vi "MP-Registry.vi"(6 "Action":T18 caption="Action (def: Read)", 7 "Micropulse # In":i32, 8 "error in (no error)":errorcluster, 10 "Data in":variant) -> (0 "error out":errorcluster, 2 "Micropulse Data":T2={"Instrument Type"=enum."MicroPulse 5", "Serial #"=0, "Sample Frequency"=enum."100MHz", "dt (us)"=0.0, "DOF"=enum."8-bit Mode", "Material Velocity"=1.0, "Asynch Reads"=enum."Disabled", "NUM of Tests"=0, "System Details"={"System Type"=enum."MicroPulse 5", "Serial No."=0, "Channels"={"Conv"=0, "PA"=0, "Extra"=0}, "Sample Frequency"={"Default"=0, "Actual"=0}, "Software Versions"="", "Data Output Format"={"Default"=enum."8-bit Mode", "Actual"=enum."8-bit Mode"}, "Temperatures"={"System"=0, "Processor"=0, "Slave Sys"=0, "Slave Proc"=0}, "Tx Buffer Size"=0, "System Error"="", "No. of Cards"=0, "DAC Gain"=0, "Uptimes"={"since Power"=0, "since RSTS"=0, "since SRST"=0}, "Voltages"=[], "Interface Cards"=[]}, "Gates"=[], "Encoders"=[], "CMD LUT"=variant, "Command List"=""} {"System Details"."Interface Cards"."FPGA - T" format="%.0f °C"; "System Details"."Interface Cards"."Board - T" format="%.0f °C"; "System Details"."Voltages"."Difference" format="%.2fV"; "System Details"."Voltages"."Measured" format="%.2fV"; "System Details"."Voltages"."Nominal" format="%.2fV"; "System Details"."DAC Gain" format="%.0fdB"; "System Details"."Tx Buffer Size" format="%.0fMB"; "System Details"."Temperatures"."Slave Proc" format="%.0f C"; "System Details"."Temperatures"."Slave Sys" format="%.0f C"; "System Details"."Temperatures"."Processor" format="%.0f C"; "System Details"."Temperatures"."System" format="%.0f C"; "System Details"."Sample Frequency"."Actual" format="%.0fMHz"; "System Details"."Sample Frequency"."Default" format="%.0fMHz"; "Encoders"."Encoder Filter" max=255; "Encoders"."Backlash Period (s)" min=0.0005 max=10.0 step=0.0005; "Encoders"."Multiplier" min=1 max=100000; "Encoders"."Counts/mm" min=1 max=100000; "Gates"."Insp Gates"."Max # Peaks" max=64000 step=100; "Gates"."Insp Gates"."Threshold" min=10 max=4095 step=10; "Gates"."Insp Gates"."Length (us)" min=0.0 max=96000.0 step=100.0; "Gates"."Insp Gates"."Start (us)" min=0.0 max=64000.0 step=100.0; "Gates"."Echo Gate"."Threshold" min=10 max=4095 step=10; "Gates"."Echo Gate"."Length (us)" min=0.0 max=96000.0 step=100.0; "Gates"."Echo Gate"."Start (us)" min=0.0 max=64000.0 step=100.0; "Gates"."Display Gate"."Length" min=0.0 max=64000.0 step=1000.0; "Gates"."Display Gate"."Start" min=0.0 max=64000.0 step=1000.0}, 3 "TCP config":T1={"Connection ID"=refnum, "IP address"="10.1.1.2", "host port"=1067, "OC timeout"=-1, "Read timeout"=0, "Write timeout"=0} {"Write timeout" format="%dms"; "Read timeout" format="%dms"; "OC timeout" format="%dms"}, 5 "Micropulse # Out":i32)   [LabVIEW 2026, in "MicroPulse_Driver.lvlib"]
uses:
  MicroPulse_Driver.lvlib
  MP-Registry Action-Enum.ctl
  Public/Data/Datatypes/MP-Registry Data-Cluster.ctl
  <instrlib>/MicroPulse/Public/Data/Datatypes/MP - instrument type.ctl
  Public/Data/Datatypes/MP - sample frequency.ctl
  Public/Data/Datatypes/MP - data output format.ctl
  Public/Data/Datatypes/MP - asynch read mode.ctl
  Public/Data/Datatypes/MP - general system status.ctl
  Public/Data/Datatypes/MP - interface card status.ctl
  Public/Data/Datatypes/subdatatypes/MP - Registry Gates.ctl
  Public/Data/Datatypes/MP - display gate.ctl
  Public/Data/Datatypes/MP - echo gate mode.ctl
  Public/Data/Datatypes/MP - echo gate parameters.ctl
  Public/Data/Datatypes/MP - multigate inspection gate parameters.ctl
  Public/Data/Datatypes/MP - hysteresis level.ctl
  Public/Data/Datatypes/MP - multigate mode.ctl
  Public/Data/Datatypes/MP - encoder settings.ctl
  Public/Data/Datatypes/MP - encoder type.ctl
  Public/Data/Datatypes/TCP config.ctl
panel:
  out "All Micropulse Data":T2[](array[typedef]) {"System Details"."Interface Cards"."FPGA - T" format="%.0f °C"; "System Details"."Interface Cards"."Board - T" format="%.0f °C"; "System Details"."Voltages"."Difference" format="%.2fV"; "System Details"."Voltages"."Measured" format="%.2fV"; "System Details"."Voltages"."Nominal" format="%.2fV"; "System Details"."DAC Gain" format="%.0fdB"; "System Details"."Tx Buffer Size" format="%.0fMB"; "System Details"."Temperatures"."Slave Proc" format="%.0f C"; "System Details"."Temperatures"."Slave Sys" format="%.0f C"; "System Details"."Temperatures"."Processor" format="%.0f C"; "System Details"."Temperatures"."System" format="%.0f C"; "System Details"."Sample Frequency"."Actual" format="%.0fMHz"; "System Details"."Sample Frequency"."Default" format="%.0fMHz"; "Encoders"."Encoder Filter" max=255; "Encoders"."Backlash Period (s)" min=0.0005 max=10.0 step=0.0005; "Encoders"."Multiplier" min=1 max=100000; "Encoders"."Counts/mm" min=1 max=100000; "Gates"."Insp Gates"."Max # Peaks" max=64000 step=100; "Gates"."Insp Gates"."Threshold" min=10 max=4095 step=10; "Gates"."Insp Gates"."Length (us)" min=0.0 max=96000.0 step=100.0; "Gates"."Insp Gates"."Start (us)" min=0.0 max=64000.0 step=100.0; "Gates"."Echo Gate"."Threshold" min=10 max=4095 step=10; "Gates"."Echo Gate"."Length (us)" min=0.0 max=96000.0 step=100.0; "Gates"."Echo Gate"."Start (us)" min=0.0 max=64000.0 step=100.0; "Gates"."Display Gate"."Length" min=0.0 max=64000.0 step=1000.0; "Gates"."Display Gate"."Start" min=0.0 max=64000.0 step=1000.0}
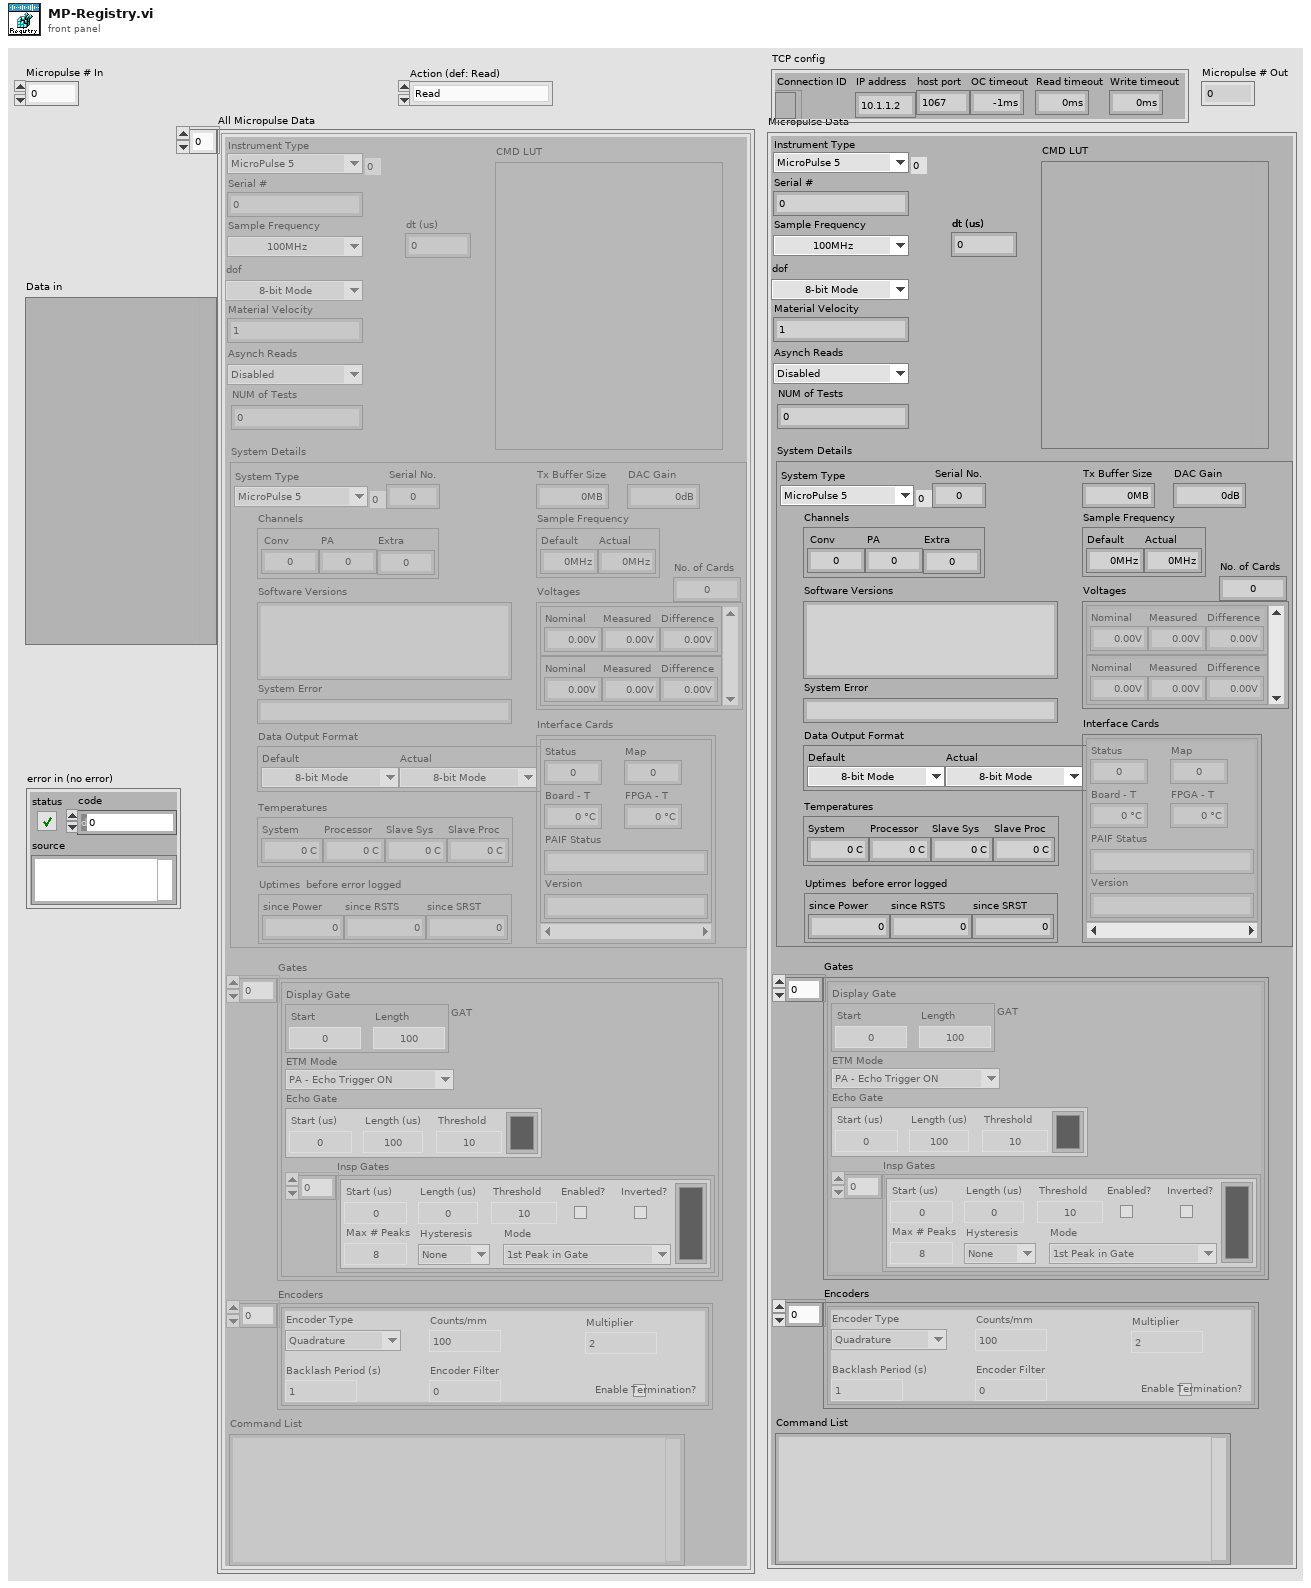
[diagram p1: front panel]
types:
  T1 = typedef "MicroPulse_Driver.lvlib/TCP config.ctl" = cluster{"Connection ID":refnum<k5>, "IP address":string, "host port":u16, "OC timeout":i32, "Read timeout":i32, "Write timeout":i32}
  T2 = typedef "MicroPulse_Driver.lvlib/MP-Registry Data-Cluster.ctl" = cluster{"Instrument Type":T3, "Serial #":u64, "Sample Frequency":T4, "dt (us)":dbl, "DOF":T5, "Material Velocity":dbl, "Asynch Reads":T6, "NUM of Tests":u32, "System Details":T7, "Gates":T9[], "Encoders":T16[], "CMD LUT":variant, "Command List":string}
  T3 = typedef "MicroPulse_Driver.lvlib/MP - instrument type.ctl" = enum16{"MicroPulse 5", "LT1", "LT2", "LTPA", "MPLT", "MicroPulse 6", "PipeScanner", "<MicroPulse>", "Micropulse 4", "Simulated Data"}
  T4 = typedef "MicroPulse_Driver.lvlib/MP - sample frequency.ctl" = enum16{"Use Default", "200MHz (LT2 only)", "100MHz", "50MHz", "25MHz", "10MHz"}
  T5 = typedef "MicroPulse_Driver.lvlib/MP - data output format.ctl" = enum16{"", "8-bit Mode", "10-bit Mode", "12-bit Mode", "16-bit Mode", "8-bit Log Mode", "12-bit Packed Mode"}
  T6 = typedef "MicroPulse_Driver.lvlib/MP - asynch read mode.ctl" = enum16{"Disabled", "Enabled"}
  T7 = typedef "MicroPulse_Driver.lvlib/MP - general system status.ctl" = cluster{"System Type":T3, "Serial No.":u64, "Channels":cluster{"Conv":u8, "PA":u16, "Extra":u32}, "Sample Frequency":cluster{"Default":u8, "Actual":u8}, "Software Versions":string, "Data Output Format":cluster{"Default":T5, "Actual":T5}, "Temperatures":cluster{"System":u8, "Processor":u8, "Slave Sys":u8, "Slave Proc":u8}, "Tx Buffer Size":u32, "System Error":string, "No. of Cards":u8, "DAC Gain":i16, "Uptimes":cluster{"since Power":u32, "since RSTS":u32, "since SRST":u32}, "Voltages":cluster{"Nominal":dbl, "Measured":dbl, "Difference":dbl}[], "Interface Cards":T8[]}
  T8 = typedef "MicroPulse_Driver.lvlib/MP - interface card status.ctl" = cluster{"Status":u8, "Map":u8, "Board - T":u8, "FPGA - T":u8, "PAIF Status":string, "Version":string}
  T9 = typedef "MicroPulse_Driver.lvlib/MP - Registry Gates.ctl" = cluster{"Display Gate":T10, "ETM Mode":T11, "Echo Gate":T12, "Insp Gates":T13[]}
  T10 = typedef "MicroPulse_Driver.lvlib/MP - display gate.ctl" = cluster{"Start":dbl, "Length":dbl}
  T11 = typedef "MicroPulse_Driver.lvlib/MP - echo gate mode.ctl" = enum16{"Echo Trigger OFF", "Echo Gate Display Mode", "Echo Trigger ON", "Multi Gate or FMC Mode", "Reserved", "PA - Echo Trigger ON"}
  T12 = typedef "MicroPulse_Driver.lvlib/MP - echo gate parameters.ctl" = cluster{"Start (us)":dbl, "Length (us)":dbl, "Threshold":u16, "Colour":u32}
  T13 = typedef "MicroPulse_Driver.lvlib/MP - multigate inspection gate parameters.ctl" = cluster{"Start (us)":dbl, "Length (us)":dbl, "Threshold":u16, "Enabled?":bool, "Max # Peaks":u16, "Hysteresis":T14, "Mode":T15, "Inverted?":bool, "Colour ":u32}
  T14 = typedef "MicroPulse_Driver.lvlib/MP - hysteresis level.ctl" = enum16{"None", "3dB", "6dB", "9dB", "12dB"}
  T15 = typedef "MicroPulse_Driver.lvlib/MP - multigate mode.ctl" = enum16{"1st Peak in Gate", "Largest Peak In Gate", "All Peaks In Gate", "1st Threshold Crossing"}
  T16 = typedef "MicroPulse_Driver.lvlib/MP - encoder settings.ctl" = cluster{"Encoder Type":T17, "Counts/mm":u32, "Enable Termination?":bool, "Multiplier":u32, "Backlash Period (s)":dbl, "Encoder Filter":u32}
  T17 = typedef "MicroPulse_Driver.lvlib/MP - encoder type.ctl" = enum16{"Quadrature", "Step/Direction"}
  T18 = typedef "MicroPulse_Driver.lvlib/MP-Registry Action-Enum.ctl" = enum16{"Read", "Add Test", "Add Command", "Add Gate Command", "Add Encoder Command", "Clear Command  List", "Set Registry", "Set System Details", "Set DOF", "Set Velocity", "Disable Asynch Reads", "Enable Asynch Reads", "Add Connection", "Disconnect", "Shutdown"}
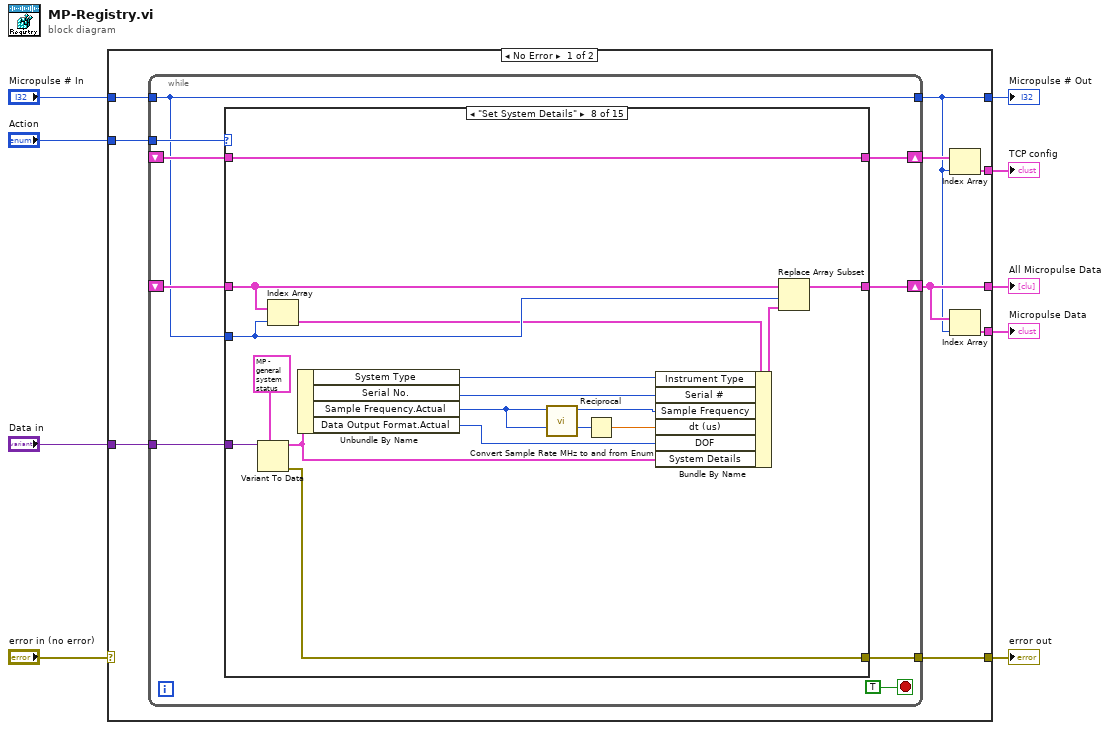
[diagram p0: block diagram]
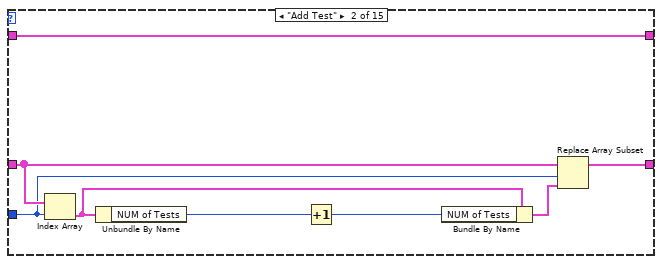
[diagram p3: hidden frame]
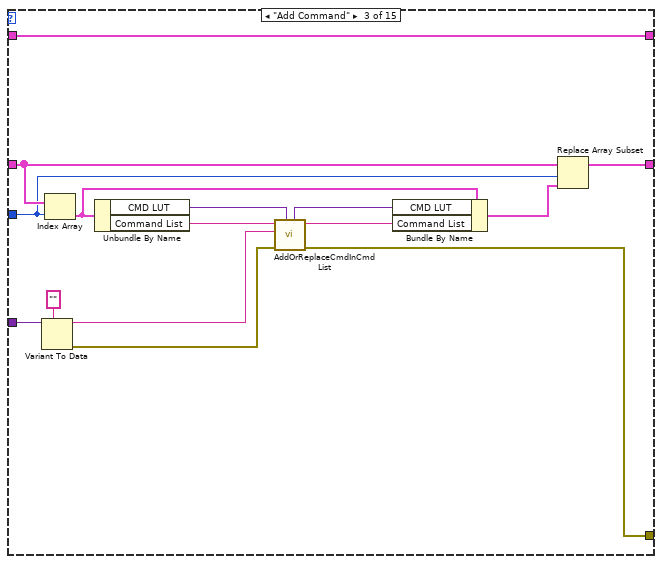
[diagram p4: hidden frame]
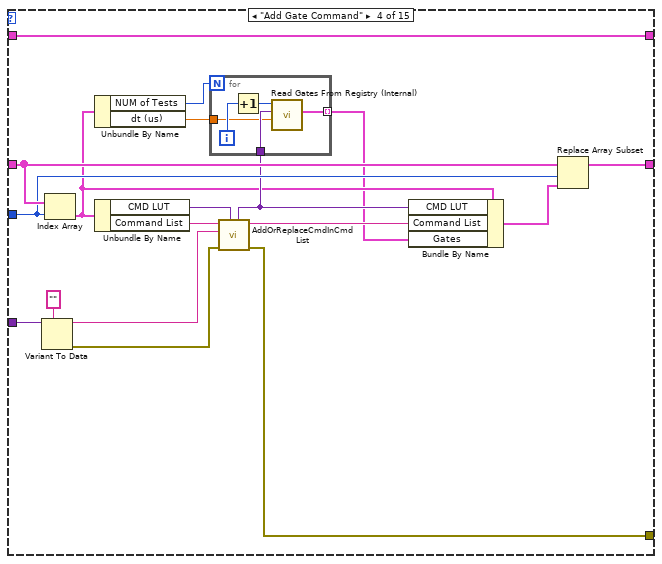
[diagram p5: hidden frame]
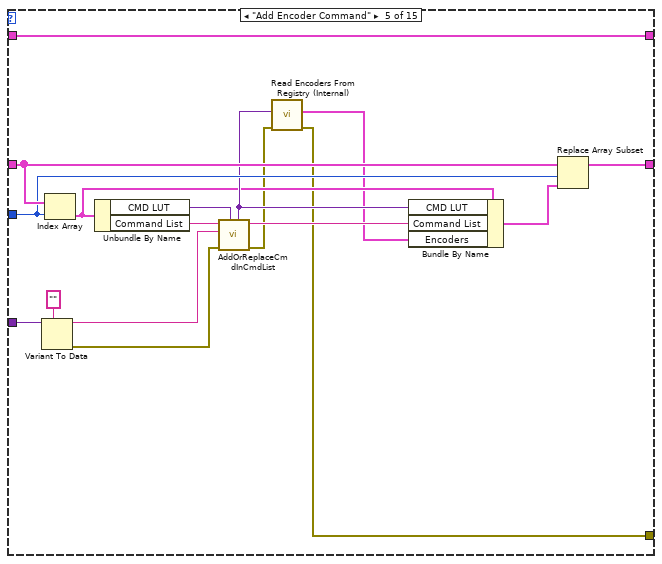
[diagram p6: hidden frame]
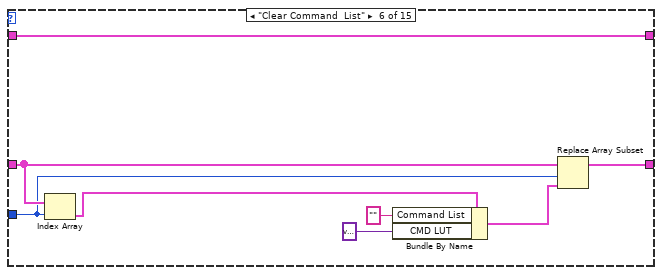
[diagram p7: hidden frame]
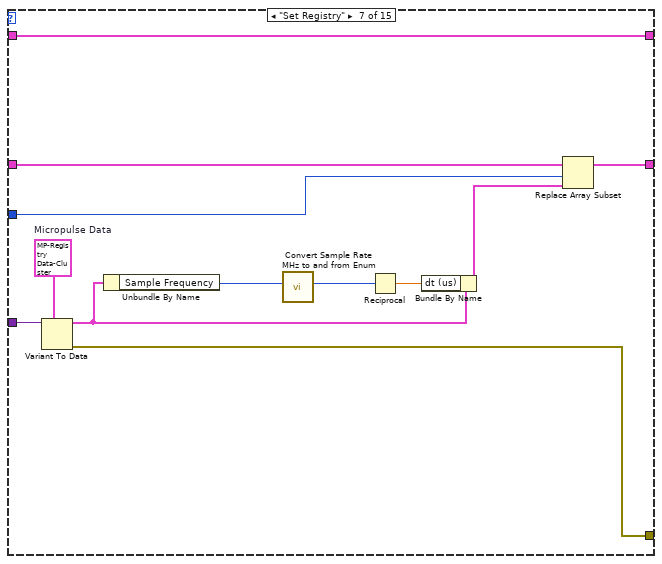
[diagram p8: hidden frame]
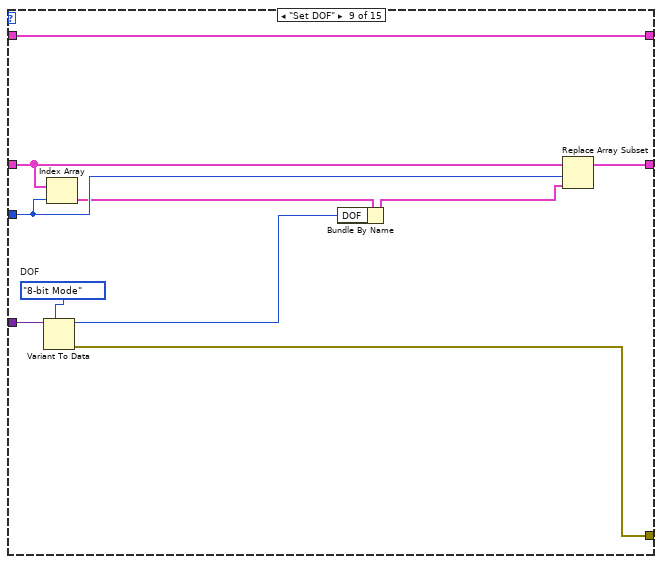
[diagram p9: hidden frame]
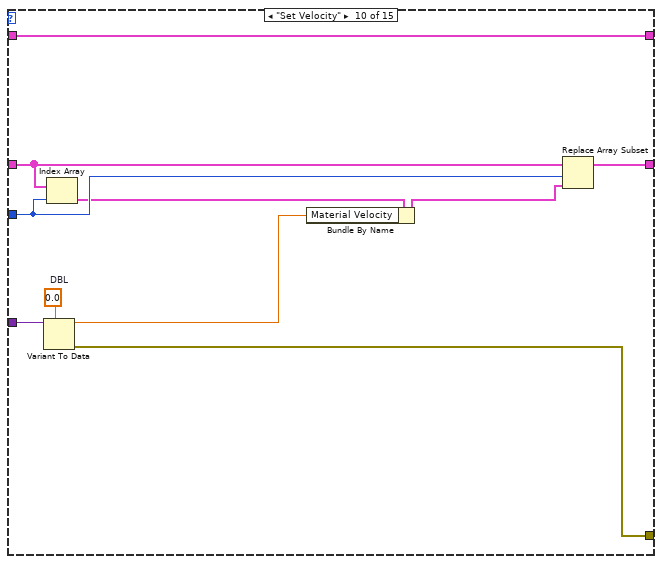
[diagram p10: hidden frame]
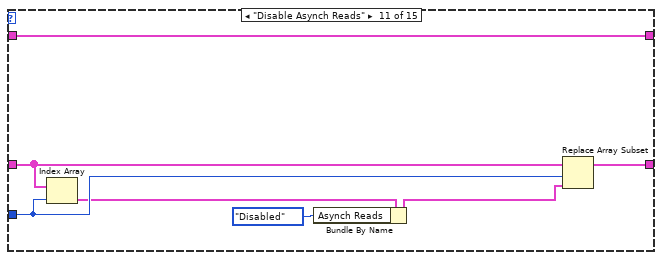
[diagram p11: hidden frame]
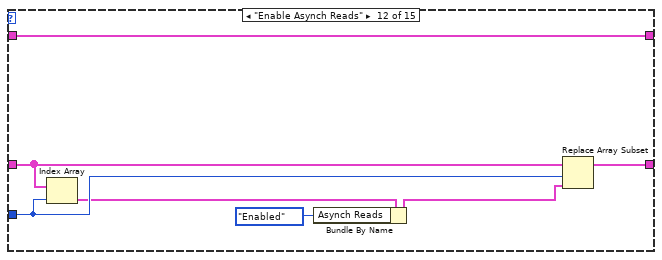
[diagram p12: hidden frame]
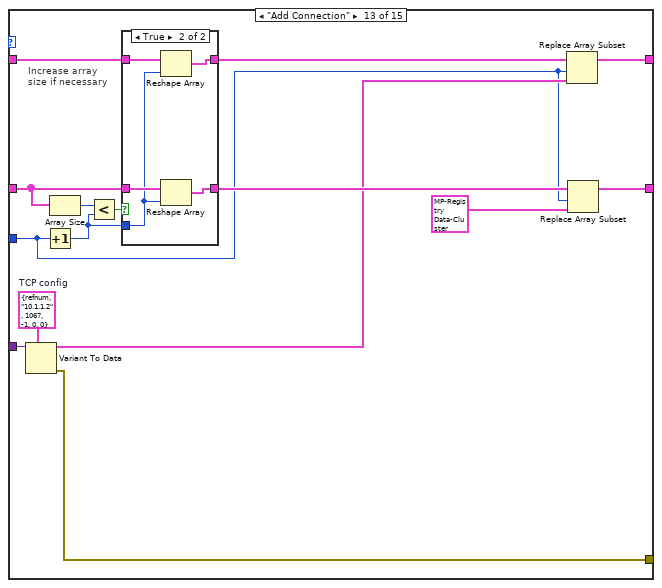
[diagram p13: hidden frame]
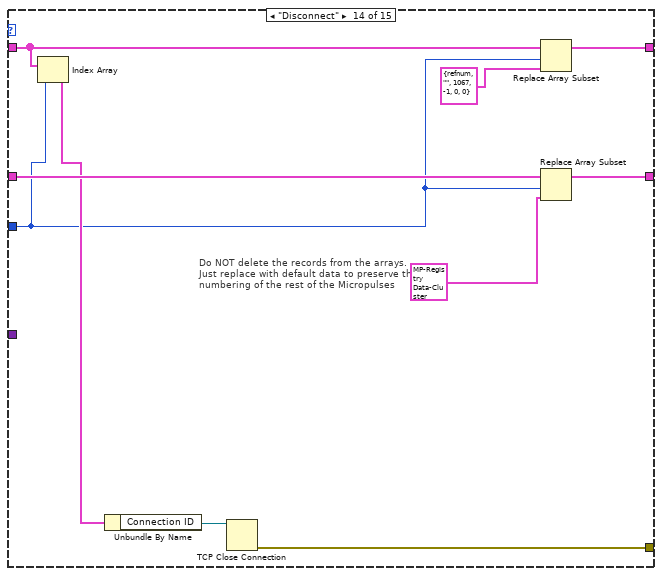
[diagram p15: hidden frame]
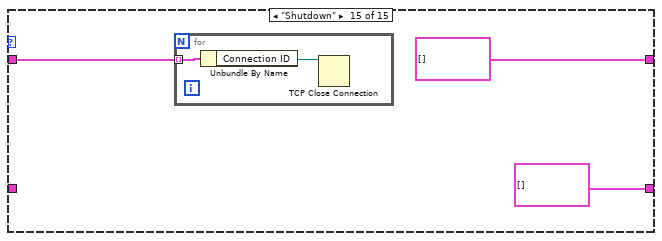
[diagram p16: hidden frame]
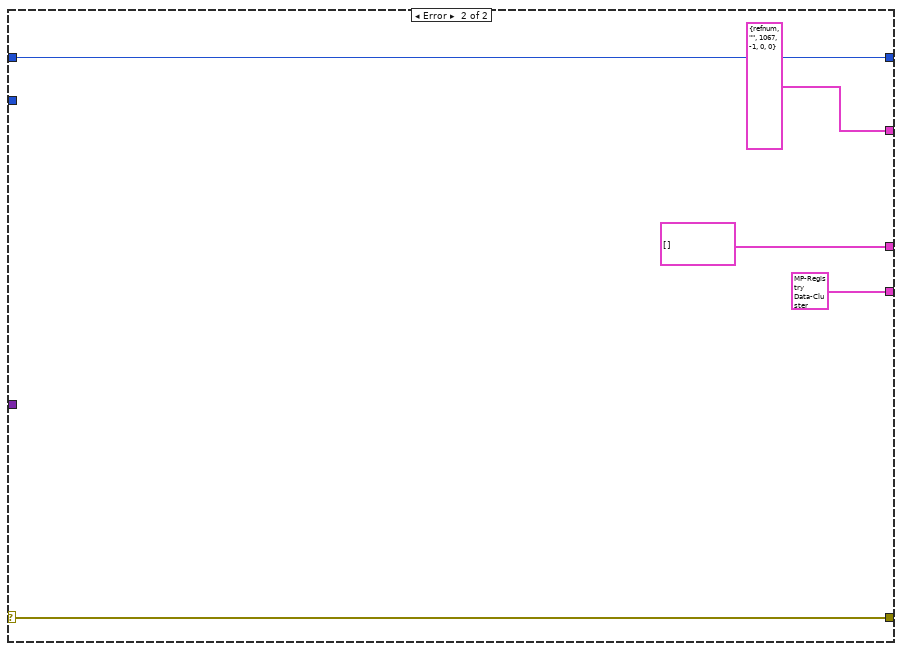
[diagram p17: hidden frame]
diagram:
  n1 = case shown="No Error" "error in (no error)" {
    selector: "error in (no error)" -> [_ w204]
    tunnel: [w12 w204] -> w8
    tunnel: "Action" -> [w18 _]
    tunnel: "Micropulse # In" -> [w16 w203]
    tunnel: [w10 w203] -> w5
    tunnel: [w15 T1 {"Connection ID"=refnum, "IP address"="", "host port"=1067, "OC timeout"=-1, "Read timeout"=0, "Write timeout"=0} ("TCP config")] -> w1
    tunnel: [w14 T2 {"Instrument Type"=enum."MicroPulse 5", "Serial #"=0, "Sample Frequency"=enum."100MHz", "dt (us)"=0.0, "DOF"=enum."8-bit Mode", "Material Velocity"=1.0, "Asynch Reads"=enum."Disabled", "NUM of Tests"=0, "System Details"={"System Type"=enum."MicroPulse 5", "Serial No."=0, "Channels"={"Conv"=0, "PA"=0, "Extra"=0}, "Sample Frequency"={"Default"=0, "Actual"=0}, "Software Versions"="", "Data Output Format"={"Default"=enum."8-bit Mode", "Actual"=enum."8-bit Mode"}, "Temperatures"={"System"=0, "Processor"=0, "Slave Sys"=0, "Slave Proc"=0}, "Tx Buffer Size"=0, "System Error"="", "No. of Cards"=0, "DAC Gain"=0, "Uptimes"={"since Power"=0, "since RSTS"=0, "since SRST"=0}, "Voltages"=[], "Interface Cards"=[]}, "Gates"=[], "Encoders"=[], "CMD LUT"=variant, "Command List"=""} ("Micropulse Data")] -> w4
    tunnel: "Data in" -> [w13 _]
    tunnel: [w11 T2[] [] ("Array")] -> w2
    frame No Error {
      n2 = while {
        shift-right: [w22] -> w11
        shift-left: _ -> [w25]
        tunnel: w18 -> [w26]
        tunnel: w16 -> [w21]
        shift-right: [w23] -> w17
        shift-left: _ -> [w24]
        tunnel: [w21] -> w10
        tunnel: w13 -> [w20]
        tunnel: [w19] -> w12
        stop <- TRUE stop-if-true
        n3 = case shown="\"Set System Details\"" w26 {
          tunnel: w21 -> [_ w34 w48 w66 w88 w97 w107 w122 w132 w143 w152 w159 w163 w185 _]
          tunnel: w25 -> [w28 w35 w50 w68 w90 w98 w111 w123 w133 w144 w153 w160 w172 w193 _]
          tunnel: w24 -> [w29 w37 w52 w70 w92 w100 w112 w128 w138 w148 w155 w162 w175 w189 w197]
          tunnel: [w29 w37 w52 w70 w92 w100 w112 w128 w138 w148 w155 w162 w168 w194 T1[] [] ("Array")] -> w23
          tunnel: [w28 w36 w51 w69 w91 w99 w110 w127 w137 w147 w154 w161 w167 w192 T2[] [] ("Array")] -> w22
          tunnel: w20 -> [_ _ w46 w64 w86 _ w109 w126 w136 w146 _ _ w170 _ _]
          tunnel: [_ _ w40 w59 w76 _ w106 w116 w134 w145 _ _ w166 w186 _] -> w19
          frame "Read", Default {
          }
          frame "Add Test" {
            n4 = Index Array(array=w35, index=w34) -> (element=w32:T2)
            n5 = Unbundle By Name(w32) -> ("NUM of Tests"=w31:u32)
            n6 = Increment(x=w31) -> (x+1=w30:u32)
            n7 = Bundle By Name(cluster=w32, "NUM of Tests"=w30) -> (w33:T2)
            n8 = Replace Array Subset(array=w35, new element=w33, index=w34) -> (w36:T2[])
          }
          frame "Add Command" {
            n9 = Variant To Data(type="", Variant=w46) -> (data=w44:string, error out=w41:errorcluster)  [unwired: 1 in]
            n10 = Index Array(array=w50, index=w48) -> (element=w42:T2)
            n11 = Unbundle By Name(w42) -> ("CMD LUT"=w39:variant, "Command List"=w49:string)
            n12 = call "AddOrReplaceCmdInCmdList.vi"("CMD LUT in"=w39, "error in (no error)"=w41, "New Command(s)"=w44, "Command List In"=w49) -> ("error out"=w40:errorcluster, "Command List Out"=w47:string, "CMD LUT out"=w38:variant)  [unwired: 5 in]
            n13 = Bundle By Name(cluster=w42, "CMD LUT"=w38, "Command List"=w47) -> (w43:T2)
            n14 = Replace Array Subset(array=w50, new element=w43, index=w48) -> (w51:T2[])
          }
          frame "Add Gate Command" {
            n15 = Variant To Data(type="", Variant=w64) -> (data=w62:string, error out=w60:errorcluster)  [unwired: 1 in]
            n16 = Index Array(array=w68, index=w66) -> (element=w56:T2)
            n17 = Unbundle By Name(w56) -> ("NUM of Tests"=w53:u32, "dt (us)"=w55:dbl)
            n18 = Unbundle By Name(w56) -> ("CMD LUT"=w58:variant, "Command List"=w67:string)
            n19 = call "AddOrReplaceCmdInCmdList.vi"("CMD LUT in"=w58, "error in (no error)"=w60, "New Command(s)"=w62, "Command List In"=w67) -> ("error out"=w59:errorcluster, "Command List Out"=w65:string, "CMD LUT out"=w57:variant)  [unwired: 5 in]
            n20 = for {
              N: w53 -> [_]
              tunnel: w57 -> [w73]
              tunnel: w55 -> [w72]
              tunnel: [w71] -> w54 mode=indexing
              i -> [w75]
              n21 = Increment(x=w75) -> (x+1=w74:i32)
              n22 = call "Read Gates From Registry (Internal).vi"("dt (us)"=w72, "CMD LUT"=w73, "Test No."=w74) -> ("Gates"=w71:T9)  [unwired: 7 in, 1 out]
            }
            n23 = Bundle By Name(cluster=w56, "CMD LUT"=w57, "Command List"=w65, "Gates"=w54) -> (w61:T2)
            n24 = Replace Array Subset(array=w68, new element=w61, index=w66) -> (w69:T2[])
          }
          frame "Add Encoder Command" {
            n25 = Variant To Data(type="", Variant=w86) -> (data=w84:string, error out=w82:errorcluster)  [unwired: 1 in]
            n26 = Index Array(array=w90, index=w88) -> (element=w79:T2)
            n27 = Unbundle By Name(w79) -> ("CMD LUT"=w81:variant, "Command List"=w89:string)
            n28 = call "AddOrReplaceCmdInCmdList.vi"("CMD LUT in"=w81, "error in (no error)"=w82, "New Command(s)"=w84, "Command List In"=w89) -> ("error out"=w77:errorcluster, "Command List Out"=w87:string, "CMD LUT out"=w80:variant)  [unwired: 5 in]
            n29 = call "Read Encoders From Registry (Internal).vi"("error in (no error)"=w77, "CMD LUT"=w80) -> ("error out"=w76:errorcluster, "Encoders"=w78:T16[])  [unwired: 8 in]
            n30 = Bundle By Name(cluster=w79, "CMD LUT"=w80, "Command List"=w87, "Encoders"=w78) -> (w83:T2)
            n31 = Replace Array Subset(array=w90, new element=w83, index=w88) -> (w91:T2[])
          }
          frame "Clear Command  List" {
            n32 = Index Array(array=w98, index=w97) -> (element=w95:T2)
            n33 = Bundle By Name(cluster=w95, "Command List"="", "CMD LUT"=variant) -> (w96:T2)
            n34 = Replace Array Subset(array=w98, new element=w96, index=w97) -> (w99:T2[])
          }
          frame "Set Registry" {
            w108 = T2 {"Instrument Type"=enum."MicroPulse 5", "Serial #"=0, "Sample Frequency"=enum."100MHz", "dt (us)"=0.0, "DOF"=enum."8-bit Mode", "Material Velocity"=1.0, "Asynch Reads"=enum."Disabled", "NUM of Tests"=0, "System Details"={"System Type"=enum."MicroPulse 5", "Serial No."=0, "Channels"={"Conv"=0, "PA"=0, "Extra"=0}, "Sample Frequency"={"Default"=0, "Actual"=0}, "Software Versions"="", "Data Output Format"={"Default"=enum."8-bit Mode", "Actual"=enum."8-bit Mode"}, "Temperatures"={"System"=0, "Processor"=0, "Slave Sys"=0, "Slave Proc"=0}, "Tx Buffer Size"=0, "System Error"="", "No. of Cards"=0, "DAC Gain"=0, "Uptimes"={"since Power"=0, "since RSTS"=0, "since SRST"=0}, "Voltages"=[], "Interface Cards"=[]}, "Gates"=[], "Encoders"=[], "CMD LUT"=variant, "Command List"=""}  # Micropulse Data
            n35 = Variant To Data(type=w108, Variant=w109) -> (data=w105:T2, error out=w106:errorcluster)  [unwired: 1 in]
            n36 = Unbundle By Name(w105) -> ("Sample Frequency"=w102:T4)
            n37 = call "Convert Sample Rate MHz to and from Enum.vi"("Sample Frequency enum in"=w102) -> ("MHz out"=w101:u8)  [unwired: 9 in, 1 out]
            n38 = Reciprocal(x=w101) -> (1/x=w103:dbl)
            n39 = Bundle By Name(cluster=w105, "dt (us)"=w103) -> (w104:T2)
            n40 = Replace Array Subset(array=w111, new element=w104, index=w107) -> (w110:T2[])
          }
          frame "Set System Details" {
            n41 = Variant To Data(type=T7 {"System Type"=enum."MicroPulse 5", "Serial No."=0, "Channels"={"Conv"=0, "PA"=0, "Extra"=0}, "Sample Frequency"={"Default"=0, "Actual"=0}, "Software Versions"="", "Data Output Format"={"Default"=enum."8-bit Mode", "Actual"=enum."8-bit Mode"}, "Temperatures"={"System"=0, "Processor"=0, "Slave Sys"=0, "Slave Proc"=0}, "Tx Buffer Size"=0, "System Error"="", "No. of Cards"=0, "DAC Gain"=0, "Uptimes"={"since Power"=0, "since RSTS"=0, "since SRST"=0}, "Voltages"=[], "Interface Cards"=[]} ("System Details"), Variant=w126) -> (data=w118:T7, error out=w116:errorcluster)  [unwired: 1 in]
            n42 = Index Array(array=w123, index=w122) -> (element=w121:T2)
            n43 = Unbundle By Name(w118) -> ("System Type"=w117:T3, "Serial No."=w120:u64, "Sample Frequency.Actual"=w114:u8, "Data Output Format.Actual"=w119:T5)
            n44 = call "Convert Sample Rate MHz to and from Enum.vi"("MHz in"=w114) -> ("Sample Frequency enum out"=w113:T4)  [unwired: 9 in, 1 out]
            n45 = Reciprocal(x=w114) -> (1/x=w115:dbl)
            n46 = Bundle By Name(cluster=w121, "Instrument Type"=w117, "Serial #"=w120, "Sample Frequency"=w113, "dt (us)"=w115, "DOF"=w119, "System Details"=w118) -> (w125:T2)
            n47 = Replace Array Subset(array=w123, new element=w125, index=w122) -> (w127:T2[])
          }
          frame "Set DOF" {
            w135 = MP_-_data_output_format."8-bit Mode"  # DOF
            n48 = Variant To Data(type=w135, Variant=w136) -> (data=w129:T5, error out=w134:errorcluster)  [unwired: 1 in]
            n49 = Index Array(array=w133, index=w132) -> (element=w131:T2)
            n50 = Bundle By Name(cluster=w131, "DOF"=w129) -> (w130:T2)
            n51 = Replace Array Subset(array=w133, new element=w130, index=w132) -> (w137:T2[])
          }
          frame "Set Velocity" {
            w139 = 0.0  # DBL
            n52 = Variant To Data(type=w139, Variant=w146) -> (data=w140:dbl, error out=w145:errorcluster)  [unwired: 1 in]
            n53 = Index Array(array=w144, index=w143) -> (element=w142:T2)
            n54 = Bundle By Name(cluster=w142, "Material Velocity"=w140) -> (w141:T2)
            n55 = Replace Array Subset(array=w144, new element=w141, index=w143) -> (w147:T2[])
          }
          frame "Disable Asynch Reads" {
            n56 = Index Array(array=w153, index=w152) -> (element=w151:T2)
            n57 = Bundle By Name(cluster=w151, "Asynch Reads"=MP_-_asynch_read_mode."Disabled") -> (w150:T2)
            n58 = Replace Array Subset(array=w153, new element=w150, index=w152) -> (w154:T2[])
          }
          frame "Enable Asynch Reads" {
            n59 = Index Array(array=w160, index=w159) -> (element=w158:T2)
            n60 = Bundle By Name(cluster=w158, "Asynch Reads"=MP_-_asynch_read_mode."Enabled") -> (w157:T2)
            n61 = Replace Array Subset(array=w160, new element=w157, index=w159) -> (w161:T2[])
          }
          frame "Add Connection" {
            w169 = T1 {"Connection ID"=refnum, "IP address"="10.1.1.2", "host port"=1067, "OC timeout"=-1, "Read timeout"=0, "Write timeout"=0}  # TCP config
            # "Increase array\nsize if necessary"
            n62 = Variant To Data(type=w169, Variant=w170) -> (data=w165:T1, error out=w166:errorcluster)  [unwired: 1 in]
            n63 = Increment(x=w163) -> (x+1=w173:i32)
            n64 = Array Size(array=w172) -> (size(s)=w177:i32)
            n65 = Less?(x=w177, y=w173) -> (x < y?=w176:bool)
            n66 = case shown="True" w176 {
              tunnel: w175 -> [w179 w184]
              tunnel: [w179 w183] -> w174
              tunnel: w173 -> [_ w180]
              tunnel: w172 -> [w178 w182]
              tunnel: [w178 w181] -> w171
              frame False {
              }
              frame True {
                n67 = Reshape Array(w184, w180) -> (w183:T1[])
                n68 = Reshape Array(w182, w180) -> (w181:T2[])
              }
            }
            n69 = Replace Array Subset(array=w174, new element=w165, index=w163) -> (w168:T1[])
            n70 = Replace Array Subset(array=w171, new element=T2 {"Instrument Type"=enum."<MicroPulse>", "Serial #"=0, "Sample Frequency"=enum."100MHz", "dt (us)"=0.0, "DOF"=enum."8-bit Mode", "Material Velocity"=1.0, "Asynch Reads"=enum."Disabled", "NUM of Tests"=0, "System Details"={"System Type"=enum."MicroPulse 5", "Serial No."=0, "Channels"={"Conv"=0, "PA"=0, "Extra"=0}, "Sample Frequency"={"Default"=0, "Actual"=0}, "Software Versions"="", "Data Output Format"={"Default"=enum."8-bit Mode", "Actual"=enum."8-bit Mode"}, "Temperatures"={"System"=0, "Processor"=0, "Slave Sys"=0, "Slave Proc"=0}, "Tx Buffer Size"=0, "System Error"="", "No. of Cards"=0, "DAC Gain"=0, "Uptimes"={"since Power"=0, "since RSTS"=0, "since SRST"=0}, "Voltages"=[], "Interface Cards"=[]}, "Gates"=[], "Encoders"=[], "CMD LUT"=variant, "Command List"=""} ("new element/subarray"), index=w163) -> (w167:T2[])
          }
          frame "Disconnect" {
            # "Do NOT delete the records from the arrays.\nJust replace with default data to preserve the\nnumbering of the rest of the Micropulses"
            n71 = Index Array(array=w189, index=w185) -> (element=w188:T1)
            n72 = Unbundle By Name(w188) -> ("Connection ID"=w187:refnum<k5>)
            n73 = TCP Close Connection(connection ID=w187) -> (error out=w186:errorcluster)  [unwired: 2 in, 1 out]
            n74 = Replace Array Subset(array=w189, new element=T1 {"Connection ID"=refnum, "IP address"="", "host port"=1067, "OC timeout"=-1, "Read timeout"=0, "Write timeout"=0} ("new element/subarray"), index=w185) -> (w194:T1[])
            n75 = Replace Array Subset(array=w193, new element=T2 {"Instrument Type"=enum."<MicroPulse>", "Serial #"=0, "Sample Frequency"=enum."100MHz", "dt (us)"=0.0, "DOF"=enum."8-bit Mode", "Material Velocity"=1.0, "Asynch Reads"=enum."Disabled", "NUM of Tests"=0, "System Details"={"System Type"=enum."MicroPulse 5", "Serial No."=0, "Channels"={"Conv"=0, "PA"=0, "Extra"=0}, "Sample Frequency"={"Default"=0, "Actual"=0}, "Software Versions"="", "Data Output Format"={"Default"=enum."8-bit Mode", "Actual"=enum."8-bit Mode"}, "Temperatures"={"System"=0, "Processor"=0, "Slave Sys"=0, "Slave Proc"=0}, "Tx Buffer Size"=0, "System Error"="", "No. of Cards"=0, "DAC Gain"=0, "Uptimes"={"since Power"=0, "since RSTS"=0, "since SRST"=0}, "Voltages"=[], "Interface Cards"=[]}, "Gates"=[], "Encoders"=[], "CMD LUT"=variant, "Command List"=""} ("new element/subarray"), index=w185) -> (w192:T2[])
          }
          frame "Shutdown" {
            n76 = for {
              tunnel: w197 -> [w199] mode=indexing
              n77 = Unbundle By Name(w199) -> ("Connection ID"=w198:refnum<k5>)
              n78 = TCP Close Connection(connection ID=w198) -> ()  [unwired: 2 in, 2 out]
            }
          }
        }
      }
      n79 = Index Array(array=w17, index=w10) -> (element=w15:T1)
      n80 = Index Array(array=w11, index=w10) -> (element=w14:T2)
    }
    frame Error {
    }
  }
  "error out" <- w8
  "Micropulse # Out" <- w5
  "Micropulse Data" <- w4
  "All Micropulse Data" <- w2
  "TCP config" <- w1
